vi "全局变量.vi"() -> ()   [LabVIEW 2018]
uses:
  <vilib>/vision/Image Controls.llb/IMAQ Image.ctl
panel:
  out "默认标定图":T1
  out "标准标定图":T1
  out "展开图":T1
  out "实际玩轮廓与拟合外轮廓间距":dbl[](array[numeric])
  out "实际外轮廓曲率":dbl[](array[numeric])
  out "实际内轮廓与拟合内轮廓间距":dbl[](array[numeric])
  out "实际内轮廓曲率":dbl[](array[numeric])
  in  "Y轴像素标定值":dbl
  in  "X轴像素标定值":dbl
  out "内轮廓半径":dbl
  out "内轮廓Y":dbl
  out "内轮廓X":dbl
  out "外轮廓半径":dbl
  out "外轮廓X":dbl
  out "外轮廓Y":dbl
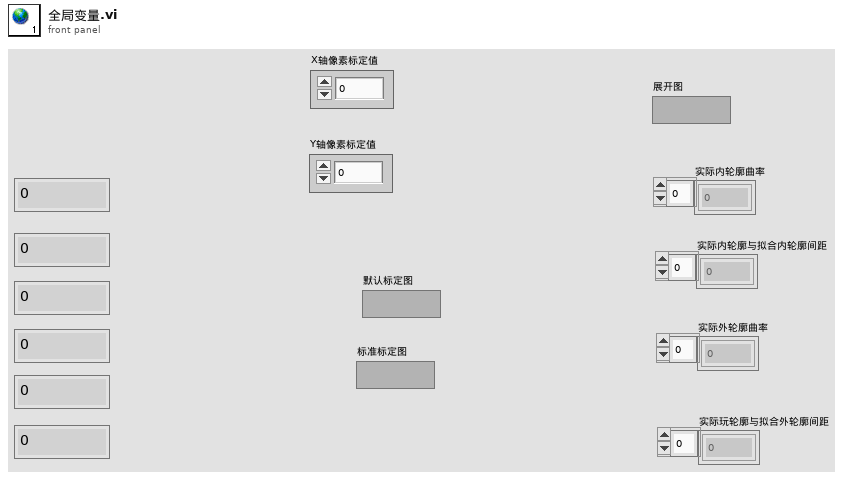
[diagram p1: front panel]
types:
  T1 = typedef "IMAQ Image.ctl" = refnum<image>
diagram:
